vi "Set Pump Fow Rate.vi"(8 "Error In":errorcluster, 9 "Pulse Width":i32, 10 "Voltage":i32, 11 "ECU COM Port":refnum<visa-resource-name>) -> (0 "Error Out":errorcluster, 3 "ECU COM Port Out":refnum<visa-resource-name>)   [LabVIEW 2017]
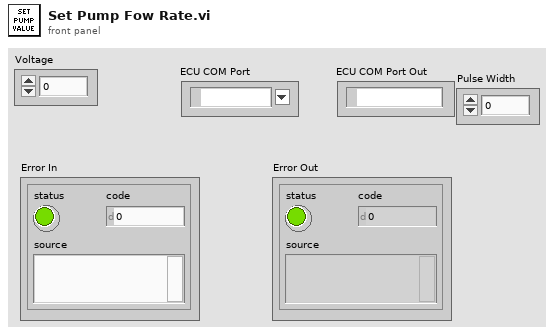
[diagram p1: front panel]
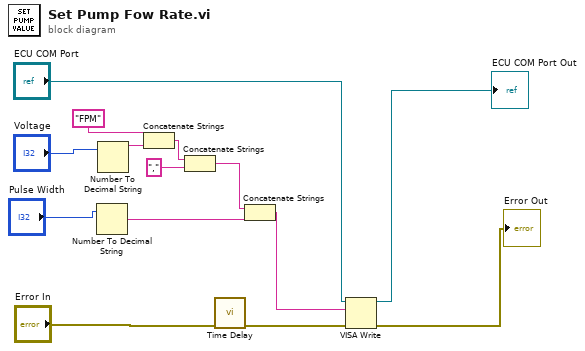
[diagram p0: block diagram]
diagram:
  n1 = Number To Decimal String(number="Pulse Width") -> (decimal integer string=w2:string)  [unwired: 1 in]
  n2 = Number To Decimal String(number="Voltage") -> (decimal integer string=w14:string)  [unwired: 1 in]
  n3 = Concatenate Strings("FPM" ("write buffer"), w14) -> (w6:string)
  n4 = Concatenate Strings(w6, "," ("write buffer")) -> (w3:string)
  n5 = call "Time Delay"("error in (no error)"="Error In") -> ("error out"=w7:errorcluster)  [unwired: 10 in]
  n6 = Concatenate Strings(w3, w2) -> (w1:string)
  n7 = VISA Write(VISA resource name="ECU COM Port", write buffer=w1, error in (no error)=w7) -> (VISA resource name out=→"ECU COM Port Out":refnum<visa-resource-name>, error out=→"Error Out":errorcluster)  [unwired: 1 out]
